vi "Configure Burst.vi"(4 "Burst Period (1 s)":dbl=1.0 min=0.002 max=1000000.0 format="%.6f", 6 "Burst Count (1)":i32=1, 7 "Burst Mode (0: Triggered)":u16(ring) items=["Triggered", "Gated"], 8 "error in (no error)":errorcluster, 9 "Burst Phase (0 deg)":i32 min=-360 max=360, 10 "Enable Burst (T: Enable)":bool=TRUE, 11 "VISA resource name":refnum<visa-resource-name>) -> (0 "error out":errorcluster, 3 "VISA resource name out":refnum<visa-resource-name>)   [LabVIEW 2012, in "Agilent 33XXX Series.lvlib"]
doc: "Allows and configures burst. Configures the function generator to output a waveform with specified number of cycles, called burst. The carrier waveform shape and parameters are set by Configure Standard Waveform.\n\nNote:\n(1) Before using this mode, all other modes must be turned off.\n(2) This VI is valid in 33210, 33220, and 33250."
uses:
  Agilent 33XXX Series.lvlib
panel:
  # "Triggered BM Settings"
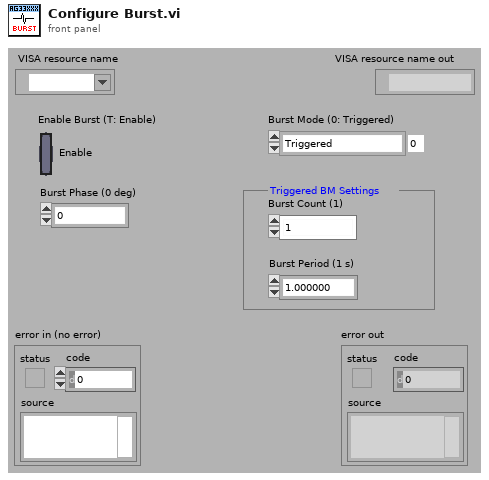
[diagram p1: front panel]
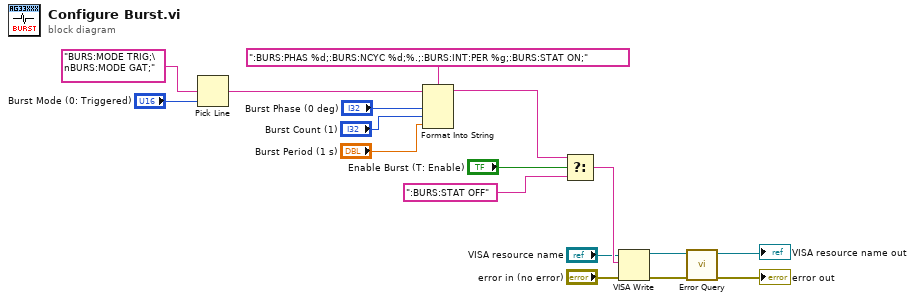
[diagram p0: block diagram]
diagram:
  n1 = Pick Line(multi-line string="BURS:MODE TRIG;\nBURS:MODE GAT;" ("f"), line index="Burst Mode (0: Triggered)") -> (output string=w6:string)  [unwired: 1 in]
  n2 = Format Into String(format string=":BURS:PHAS %d;:BURS:NCYC %d;%.;:BURS:INT:PER %g;:BURS:STAT ON;", initial string=w6, "Burst Phase (0 deg)", "Burst Count (1)", "Burst Period (1 s)") -> (resulting string=w5:string)  [unwired: 1 in, 1 out]
  n3 = Select(t=w5, s="Enable Burst (T: Enable)", f=":BURS:STAT OFF") -> (s? t:f=w4:string)
  n4 = VISA Write(VISA resource name="VISA resource name", write buffer=w4, error in (no error)="error in (no error)") -> (VISA resource name out=w17:refnum<visa-resource-name>, error out=w16:errorcluster)  [unwired: 1 out]
  n5 = call "Error Query.vi"("error in (no error)"=w16, "VISA resource name"=w17) -> ("error out"=→"error out":errorcluster, "VISA resource name out"=→"VISA resource name out":refnum<visa-resource-name>)  [unwired: 6 in, 2 out]
